vi "host_for vst high BW low frequncy.vi"() -> ()   [LabVIEW 2021]
uses:
  <vilib>/userdefined/High Color/nirio_resource_hc.ctl
  CTL/user config.ctl
  classes/p2p vst/p2p vst.lvclass
  CTL/emitter params.ctl
  CTL/mode_type.ctl
  <vilib>/Analysis/1siggen.llb/Ramp Pattern by Samples.vi
  <vilib>/Analysis/NI_AALBase.lvlib
panel:
  in  "hop rate (Hz)":dbl=5.0 format="%#_13g"
  out "error out":errorcluster={"status"=FALSE, "code"=5092, "source"="P2P reader underflow"}
  in  "Done Tx secenario?":bool
  in  "P2P sample rate":dbl=400000000.0
  in  "center frequency (Hz)":dbl=150000000.0
  in  "RF gain":dbl
  in  "Tab Control":T1(tab)
  in  "devicess":T2[](array[typedef])=["IF_transceiver_0", "IF_transceiver_1", "IF_transceiver_2"]
  in  "frequency list":dbl[](array[numeric])=[120000000.0, 250000000.0, 50000000.0, 200000000.0, 100000000.0, 300000000.0, 160000000.0, 220000000.0, 150000000.0] format="%#_6pHz"
  in  "d phase 2":dbl=1e-06
  in  "vst_device":refnum<k15>[](array[refnum])=["VST_5840"]
  out "dds free":bool[][](array[boolean])=[[FALSE], [TRUE], [TRUE], [TRUE], [TRUE], [TRUE], [TRUE], [TRUE], [TRUE], [TRUE], [TRUE], [TRUE], [TRUE], [TRUE], [TRUE], [TRUE]]
  out "secnario elapest":dbl=0.012987012987012988
  # "Tx state"
  # "Rx state"
  # "for zero put epsilon (almost zero)"
  # "1-2\n2-3\n3-1"
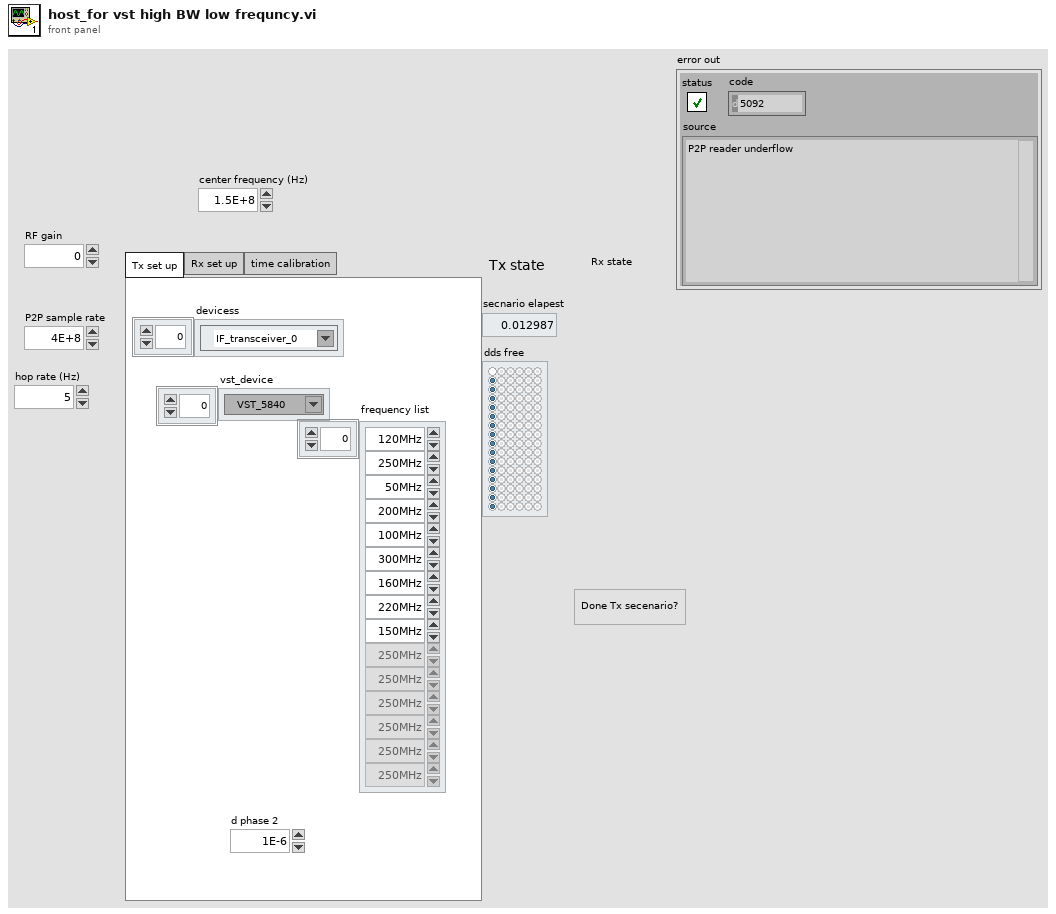
[diagram p1: front panel]
types:
  T1 = enum32{"Tx set up", "Rx set up", "time calibration"}
  T2 = typedef "nirio_resource_hc.ctl" = tag
  T3 = typedef "mode_type.ctl" = enum8{"CW", "from memory 1", "NC - cw", "LFM", "BPSK", "QPSK"}
  T4 = typedef "emitter params.ctl" = cluster{"f set":dbl[], "hop rate (Hz)":dbl, "d.c.":dbl, "amp (dB)":dbl, "mod type":T3, "mod depth":dbl, "DOA":dbl, "t start":dbl, "t end":dbl}
  T5 = typedef "user config.ctl" = cluster{"vst_device":refnum<k15>[], "RF gain ":dbl, "buffer size":u32, "center frequency (Hz) ":dbl, "P2P sample rate":dbl, "mode":enum16{"USRP - 180MHz", "5785 - 2*180MHz", "5785 - 3.2GHz", "P2P - VST"}, "devicess":T2[], "gen for df":bool, "Rx settings":cluster{"min PW         ":dbl, "max gap        ":dbl, "detection bar":dbl, "peak detect                        ":bool}, "use arb files":bool}
  T6 = typedef "PDW_lv2.ctl" = cluster{"t start":dbl, "frequency (Hz)":dbl, "duration (sec)":dbl, "amp (lin)":dbl, "mod type":T3, "mod depth":dbl, "phase (rad)":dbl[]}
  T7 = cluster{"fpga clock":dbl, "pulse transmitted":u32, "dds free":bool[][]}
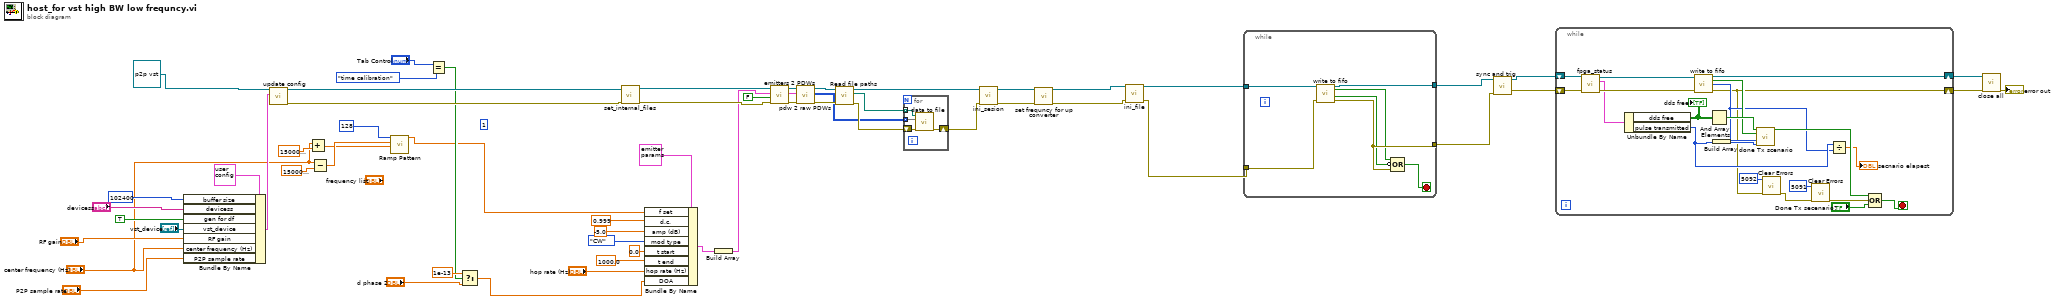
[diagram p0: block diagram]
diagram:
  (unwired) 1
  n1 = Bundle By Name(cluster=T5 {"vst_device"=["VST_1", "VST_2"], "RF gain "=10.0, "buffer size"=524288, "center frequency (Hz) "=1000000000.0, "P2P sample rate"=200000000.0, "mode"=enum."5785 - 2*180MHz", "devicess"=["IF_transiver_0", "IF_transiver_1", "IF_transiver_2"], "gen for df"=FALSE, "Rx settings"={"min PW         "=0.0, "max gap        "=0.0, "detection bar"=0.0, "peak detect                        "=FALSE}, "use arb files"=TRUE} ("user configurations"), "buffer size"=u32 102400, "devicess"="devicess", "gen for df"=TRUE, "vst_device"="vst_device", "RF gain"="RF gain", "center frequency (Hz)"="center frequency (Hz)", "P2P sample rate"="P2P sample rate") -> (w52:T5)
  n2 = call-dynamic "update config.vi"("user configurations"=w52, "p2p vst in"=refnum<class "p2p vst.lvclass"> refnum ("p2p vst.lvclass")) -> ("error out"=w59:errorcluster, "p2p vst out"=w34:refnum<class "p2p vst.lvclass">)  [unwired: 6 in, 2 out]
  n3 = Add(x="center frequency (Hz)", y=150000000.0 ("start")) -> (x+y=w2:dbl)
  n4 = Subtract(x="center frequency (Hz)", y=150000000.0 ("start")) -> (x-y=w4:dbl)
  n5 = call-poly <vilib>:"Ramp Pattern.vi"("start"=w2, "end"=w4, "samples"=128) -> ("Ramp Pattern"=w6:dbl[])  [unwired: 7 in, 1 out]
  n6 = Equal?(x="Tab Control", y=T1."time calibration") -> (x = y?=w28:bool)
  n7 = Select(t=1e-13, s=w28, f="d phase 2") -> (s? t:f=w30:dbl)
  n8 = call-dynamic "set_internal_files.vi"("error in (no error)"=w59, "device_type in"=w34) -> ("error out"=w43:errorcluster, "device_type out"=w44:refnum<class "p2p vst.lvclass">)  [unwired: 8 in]
  n9 = Bundle By Name(cluster=T4 {"f set"=[], "hop rate (Hz)"=0.0, "d.c."=0.0, "amp (dB)"=0.0, "mod type"=enum."CW", "mod depth"=0.0, "DOA"=0.0, "t start"=0.0, "t end"=0.0} ("Cluster"), "f set"=w6, "d.c."=0.999, "amp (dB)"=-5.0, "mod type"=mode_type."CW", "t start"=0.0, "t end"=1000.0, "hop rate (Hz)"="hop rate (Hz)", "DOA"=w30) -> (w9:T4)
  n10 = Build Array(w9) -> (w8:T4[])
  n11 = call-dynamic "emitters 2 PDWs.vi"("error in (no error)"=w43, "random startinig phase"=FALSE, "emmiter"=w8, "device_type in"=w44) -> ("error out"=w49:errorcluster, "sorted PDWs"=w48:T6[], "device_type out"=w47:refnum<class "p2p vst.lvclass">)  [unwired: 5 in]
  n12 = call-dynamic "pdw 2 raw PDWs.vi"("error in (no error)"=w49, "PDWs"=w48, "device_type in"=w47) -> ("error out"=w45:errorcluster, "Array"=w35:u64[][], "device_type out"=w41:refnum<class "p2p vst.lvclass">)  [unwired: 6 in]
  n13 = call-dynamic "Read file paths.vi"("error in (no error)"=w45, "device_type in"=w41) -> ("error out"=w42:errorcluster, "file paths"=w36:path[], "device_type out"=w40:refnum<class "p2p vst.lvclass">)  [unwired: 6 in, 1 out]
  n14 = for {
    tunnel: w35 -> [w61] mode=indexing
    shift-right: [w62] -> w39
    shift-left: w42 -> [w63]
    tunnel: w36 -> [w60] mode=indexing
    n15 = call "data to file.vi"("error in (no error)"=w63, "Array"=w61, "Path"=w60) -> ("error out"=w62:errorcluster)  [unwired: 8 in]
  }
  n16 = call-dynamic "ini_sesion.vi"("error in (no error)"=w39, "p2p vst in"=w40) -> ("error out"=w22:errorcluster, "p2p vst out"=w23:refnum<class "p2p vst.lvclass">)  [unwired: 8 in]
  n17 = call-dynamic "set frequncy for up converter.vi"("error in (no error)"=w22, "p2p vst in"=w23) -> ("error out"=w20:errorcluster, "p2p vst out"=w21:refnum<class "p2p vst.lvclass">)  [unwired: 8 in]
  n18 = call-dynamic "ini_file.vi"("device_type in"=w21, "error in (no error)"=w20) -> ("device_type out"=w58:refnum<class "p2p vst.lvclass">, "error out"=w57:errorcluster)  [unwired: 11 in, 1 out]
  n19 = while {
    tunnel: w58 -> [w70]
    tunnel: w57 -> [w69]
    tunnel: [w68] -> w56
    tunnel: [w66] -> w37
    stop <- w67 stop-if-true
    n20 = call-dynamic "write to fifo.vi"("p2p vst in"=w70, "error in (no error)"=w69) -> ("p2p vst out"=w68:refnum<class "p2p vst.lvclass">, "done write file"=w64:bool, "room on fifo"=w65:bool, "error out"=w66:errorcluster)  [unwired: 9 in, 1 out]
    n21 = Compound Arithmetic op=OR(w64, invert w65, w66) -> (w67:bool)
  }
  n22 = call-dynamic "sync and trig.vi"("error in (no error)"=w37, "p2p vst in"=w56) -> ("error out"=w55:errorcluster, "p2p vst out"=w38:refnum<class "p2p vst.lvclass">)  [unwired: 8 in]
  n23 = while {
    shift-right: [w87] -> w19
    shift-left: w38 -> [w89]
    shift-right: [w72] -> w18
    shift-left: w55 -> [w88]
    stop <- w80 stop-if-true
    n24 = call-dynamic "fpga_status.vi"("error in (no error)"=w88, "p2p vst in"=w89) -> ("error out"=w90:errorcluster, "pulse TX status"=w85:T7, "p2p vst out"=w91:refnum<class "p2p vst.lvclass">)  [unwired: 7 in]
    n25 = Unbundle By Name(w85) -> ("dds free"=w84:bool[][], "pulse transmitted"=w79:u32)
    "dds free" <- w84
    n26 = call-dynamic "write to fifo.vi"("p2p vst in"=w91, "error in (no error)"=w90) -> ("p2p vst out"=w87:refnum<class "p2p vst.lvclass">, "done write file"=w83:bool, "num of pulses sent to the FPGA"=w78:u32, "error out"=w72:errorcluster)  [unwired: 9 in, 1 out]
    n27 = And Array Elements(Boolean array=w84) -> (logical AND=w86:bool)
    n28 = Build Array(w79) -> (w82:u32[])
    n29 = call "done Tx scenario.vi"("all dds free"=w86, "done write files"=w83, "num of pulse sent to fpga"=w78, "pulse transmitted"=w82) -> ("Done Tx secenario?"=w81:bool)  [unwired: 11 in]
    n30 = call <vilib>:"Clear Errors.vi"("error in (no error)"=w72, "specific error code to clear (0: all)"=5092) -> ("error out"=w71:errorcluster)  [unwired: 4 in, 1 out]
    n31 = call <vilib>:"Clear Errors.vi"("error in (no error)"=w71, "specific error code to clear (0: all)"=5091) -> ("error out"=w75:errorcluster)  [unwired: 4 in, 1 out]
    n32 = Divide(x=w79, y=w78) -> (x/y=→"secnario elapest":dbl)
    n33 = Compound Arithmetic op=OR(w81, w75, "Done Tx secenario?") -> (w80:bool)
  }
  n34 = call-dynamic "close all.vi"("error in (no error)"=w18, "p2p vst in"=w19) -> ("error out"=→"error out":errorcluster)  [unwired: 8 in, 1 out]
